vi "SetHigherBound.vi"(8 "error in":errorcluster, 10 "HigherBound":timestamp, 11 "DateTimeMeasureLimit in":refnum<class "DateTimeMeasureLimit.lvclass">) -> (0 "error out":errorcluster, 3 "DateTimeMeasureLimit out":refnum<class "DateTimeMeasureLimit.lvclass">)   [LabVIEW 2021, in "ProligentXMLGenerator.lvlib" / "DateTimeMeasureLimit.lvclass"]
doc: "Real Measure Limit Higher Bound"
uses:
  DateTimeMeasureLimit.lvclass
  DateTimeMeasureLimit.lvclass/DateTimeMeasureLimit.ctl
  Base/DateTime/DateTime.lvclass
  RangeMeasureLimit/RangeMeasureLimit.lvclass
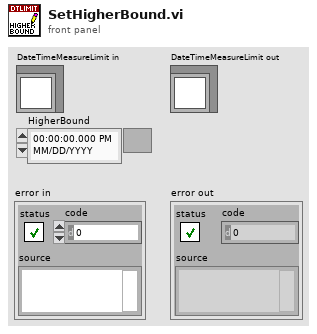
[diagram p1: front panel]
types:
  T1 = typedef "ProligentXMLGenerator.lvlib/DateTimeMeasureLimit.lvclass/Data.ctl" = cluster{"LowerBound":refnum<class "DateTime.lvclass">, "HigherBound":refnum<class "DateTime.lvclass">}
  T2 = typedef "ProligentXMLGenerator.lvlib/RangeMeasureLimit.lvclass/ComparisonType.ctl" = enum16{"LowerBound <= X <= HigherBound", "LowerBound < X <= HigherBound", "LowerBound <= X < HigherBound", "LowerBound < X < HigherBound", "LowerBound <= X", "LowerBound < X", "X <= HigherBound", "X < HigherBound", "X == HigherBound", "X != HigherBound", "X <= LowerBound OR HigherBound <= X", "X < LowerBound OR HigherBound <= X", "X <= LowerBound OR HigherBound < X", "X < LowerBound OR HigherBound < X"}
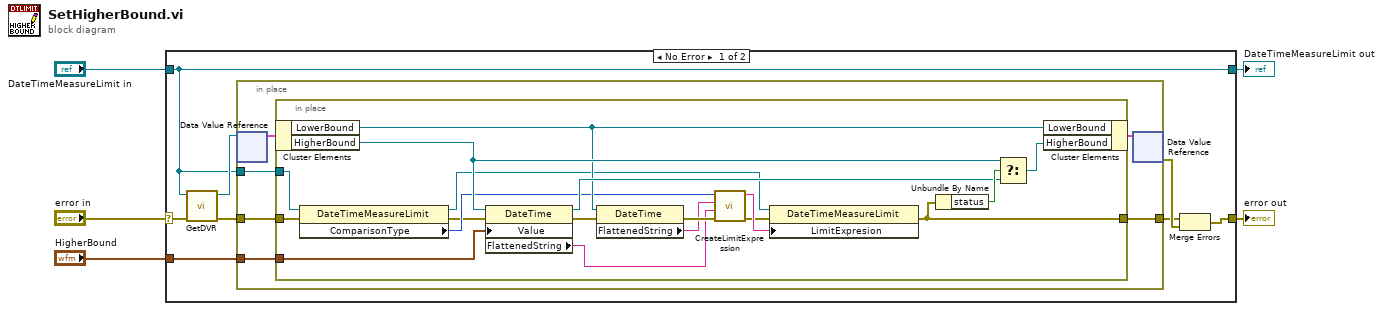
[diagram p0: block diagram]
diagram:
  n1 = case shown="No Error" "error in" {
    selector: "error in" -> [w7 w38]
    tunnel: "DateTimeMeasureLimit in" -> [w6 w39]
    tunnel: [w12 w38] -> w2
    tunnel: "HigherBound" -> [w11 _]
    tunnel: [w6 w39] -> w1
    frame No Error {
      n2 = call "GetDVR.vi"("error in"=w7, "DateTimeMeasureLimit"=w6) -> ("error out"=w10:errorcluster, "DVRReference"=w13:refnum<data-value>)  [unwired: 8 in]
      n3 = in-place "In Place Element Structure" {
        in-place-border: w11 -> [w19]
        in-place-border: w10 -> [w16]
        in-place-border: [w15] -> w8
        in-place-border: w6 -> [w14]
        n4 = in-place-dvr #1(w13) -> (w18:T1)  [unwired: 1 out]
        n5 = in-place "In Place Element Structure" {
          in-place-border: w19 -> [w32]
          in-place-border: w16 -> [w21]
          in-place-border: [w35] -> w15
          in-place-border: w14 -> [w24]
          n6 = in-place-cluster #2(w18) -> ("LowerBound"=w25:refnum<class "DateTime.lvclass">, "HigherBound"=w28:refnum<class "DateTime.lvclass">)
          n7 = property on="Property Node" class="DateTimeMeasureLimit"(reference=w24, error in=w21) -> (reference out=w22:refnum<class "DateTimeMeasureLimit.lvclass">, error out=w20:errorcluster, "ComparisonType"=w23:T2)
          n8 = property on="Property Node" class="DateTime"(reference=w28, error in=w20, "Value"=w32) -> (reference out=w26:refnum<class "DateTime.lvclass">, error out=w34:errorcluster, "FlattenedString"=w31:string)
          n9 = property on="Property Node" class="DateTime"(reference=w25, error in=w34) -> (error out=w33:errorcluster, "FlattenedString"=w30:string)  [unwired: 1 out]
          n10 = call "CreateLimitExpression.vi"("error in"=w33, "HigherBound"=w31, "LowerBound"=w30, "ComparisonType"=w23) -> ("error out"=w36:errorcluster, "LimitExpression"=w37:string)  [unwired: 6 in]
          n11 = property on="Property Node" class="DateTimeMeasureLimit"(reference=w22, error in=w36, "LimitExpresion"=w37) -> (error out=w35:errorcluster)  [unwired: 1 out]
          n12 = Unbundle By Name(w35) -> ("status"=w27:bool)
          n13 = Select(t=w28, s=w27, f=w26) -> (s? t:f=w29:refnum<class "DateTime.lvclass">)
          n14 = in-place-cluster #2("LowerBound"=w25, "HigherBound"=w29) -> (w17:T1)
        }
        n15 = in-place-dvr #1(w17) -> (w9:errorcluster)  [unwired: 1 out]
      }
      n16 = Merge Errors(w8, w9) -> (w12:errorcluster)
    }
    frame Error {
    }
  }
  "error out" <- w2
  "DateTimeMeasureLimit out" <- w1
